vi "AOchannels.vi"(8 "error in":errorcluster) -> (0 "error out":errorcluster, 3 "task out":refnum<k21>)   [LabVIEW 2013]
uses:
  <vilib>/DAQmx/create/channels.llb/DAQmx Create Channel (AO-Voltage-Basic).vi
panel:
  in  "AOchannels":tag[](array[tag])
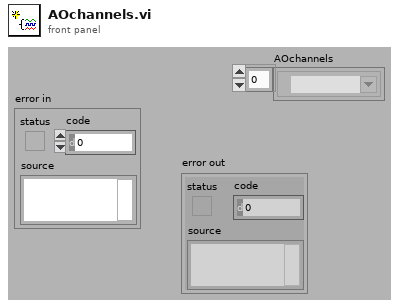
[diagram p1: front panel]
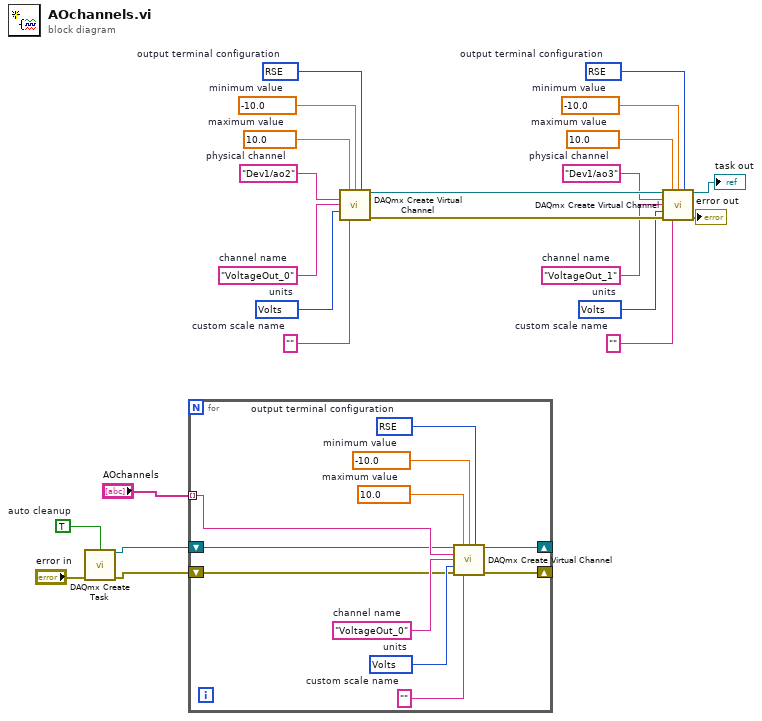
[diagram p0: block diagram]
diagram:
  w4 = 10083 items=["Default"=-1, "RSE"=10083, "Differential"=10106, "Pseudodifferential"=12529]  # output terminal configuration
  w5 = 10348 items=["Volts"=10348, "From Custom Scale"=10065]  # units
  w6 = "VoltageOut_1"  # channel name
  w9 = ""  # custom scale name
  w10 = -10.0  # minimum value
  w11 = 10.0  # maximum value
  w12 = "Dev1/ao3"  # physical channel
  w14 = 10083 items=["Default"=-1, "RSE"=10083, "Differential"=10106, "Pseudodifferential"=12529]  # output terminal configuration
  w15 = 10348 items=["Volts"=10348, "From Custom Scale"=10065]  # units
  w16 = "VoltageOut_0"  # channel name
  w18 = ""  # custom scale name
  w19 = -10.0  # minimum value
  w20 = 10.0  # maximum value
  w21 = "Dev1/ao2"  # physical channel
  w22 = TRUE  # auto cleanup
  n1 = call <vilib>:"DAQmx Create Task.vi"("auto cleanup"=w22, "error in"="error in") -> ("task out"=w2:refnum<k21>, "error out"=w1:errorcluster)  [unwired: 12 in]
  n2 = for {
    tunnel: "AOchannels" -> [w28] mode=indexing
    shift-right: [w25] -> _
    shift-left: w2 -> [w27]
    shift-right: [w24] -> _
    shift-left: w1 -> [w26]
    w34 = 10083 items=["Default"=-1, "RSE"=10083, "Differential"=10106, "Pseudodifferential"=12529]  # output terminal configuration
    w33 = 10348 items=["Volts"=10348, "From Custom Scale"=10065]  # units
    w32 = "VoltageOut_0"  # channel name
    w31 = ""  # custom scale name
    w30 = -10.0  # minimum value
    w29 = 10.0  # maximum value
    n3 = call-poly <vilib>:"DAQmx Create Virtual Channel.vi"("task in"=w27, "maximum value"=w29, "minimum value"=w30, "output terminal configuration"=w34, "physical channels"=w28, "name to assign"=w32, "units"=w33, "error in"=w26, "custom scale name"=w31) -> ("task out"=w25:refnum<k21>, "error out"=w24:errorcluster)  [unwired: 5 in]
  }
  n4 = call-poly <vilib>:"DAQmx Create Virtual Channel.vi"("maximum value"=w20, "minimum value"=w19, "output terminal configuration"=w14, "physical channels"=w21, "name to assign"=w16, "units"=w15, "custom scale name"=w18) -> ("task out"=w13:refnum<k21>, "error out"=w17:errorcluster)  [unwired: 7 in]
  n5 = call-poly <vilib>:"DAQmx Create Virtual Channel.vi"("task in"=w13, "maximum value"=w11, "minimum value"=w10, "output terminal configuration"=w4, "physical channels"=w12, "name to assign"=w6, "units"=w5, "error in"=w17, "custom scale name"=w9) -> ("task out"=→"task out":refnum<k21>, "error out"=→"error out":errorcluster)  [unwired: 5 in]
